vi "test Script EST CD.vi"(8 "error in (no error)":errorcluster, 11 "TestCase in":refnum<class "Scripting API Test Case.lvclass">) -> (0 "error out":errorcluster, 3 "TestCase out":refnum<class "Scripting API Test Case.lvclass">)   [LabVIEW 2015, in "Scripting API Test Case.lvclass"]
uses:
  Scripting API Test Case.lvclass
  Scripting API/Custom Device/Engine Simulation Toolkit Custom Device Settings.ctl
  NationalInstruments.VeriStand.SystemDefinitionAPI
  <userlib>/_OpenG.lib/file/file.llb/Append Path to Root if Relative - Scalar__ogtk.vi
  <vilib>/addons/_JKI Toolkits/VI Tester/TestCase.llb/TestCase.lvclass
  niveristand-custom-device-testing-tools/VeriStandTestUtilities/VeriStandTestUtilities.lvlib
  Scripting API/Engine Simulation Toolkit Scripting API.lvlib
panel:
  in  "Save?":bool
  out "Output Filename":string
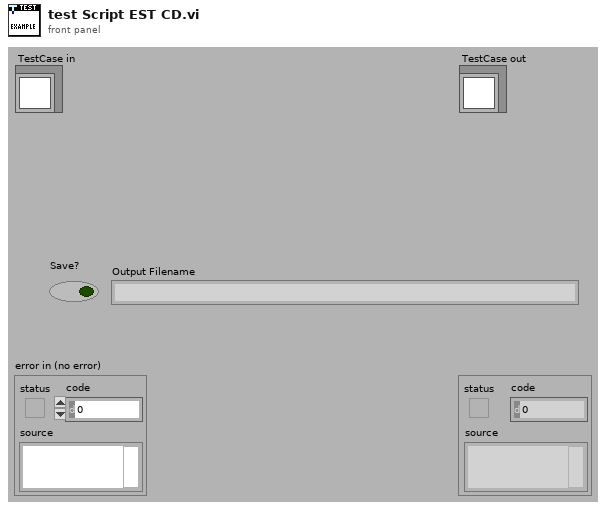
[diagram p1: front panel]
types:
  T1 = typedef "Engine Simulation Toolkit Scripting API.lvlib/Engine Simulation Toolkit Custom Device Settings.ctl" = cluster{"Name":string, "Execution priority":enum16{"Low", "Medium", "High"}, "Rate decimation":i32, "CPU":i32}
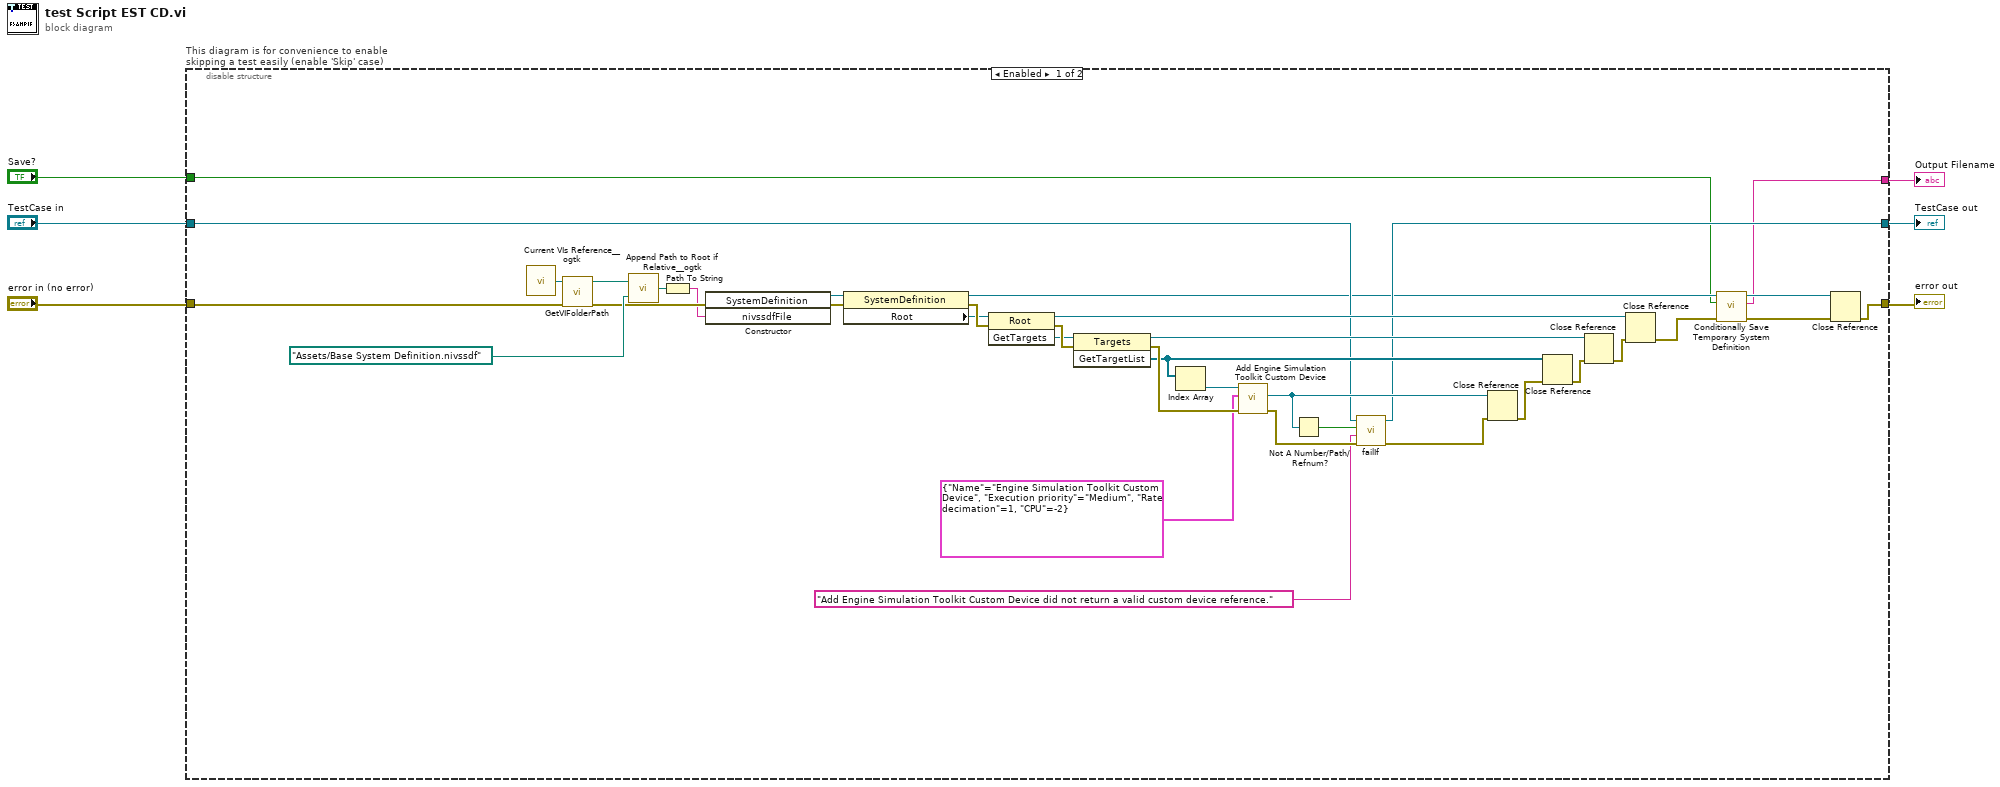
[diagram p0: block diagram]
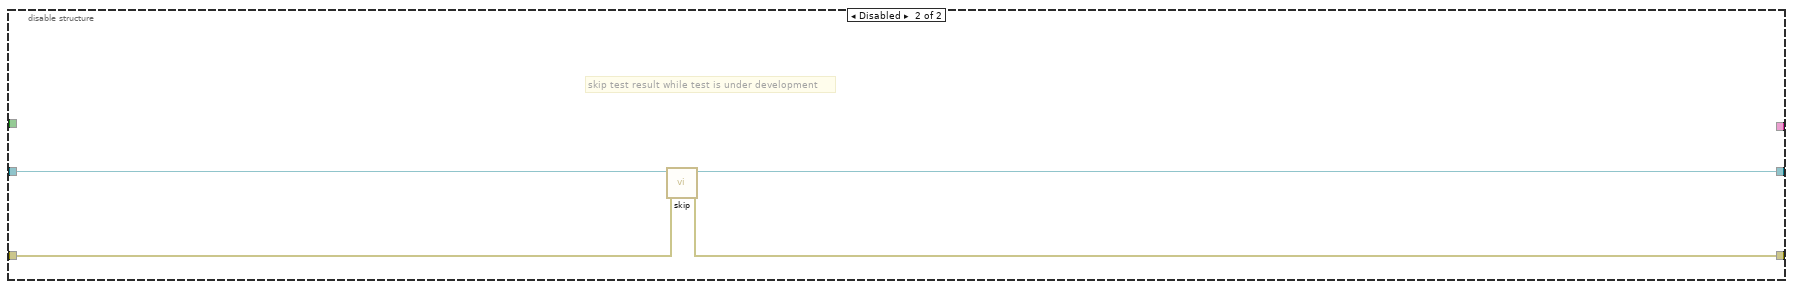
[diagram p2: hidden frame]
diagram:
  n1 = disable-structure "This diagram is for convenience to enable skipping a test easily (enable 'Skip' case)" shown="Enabled" {
    disable-tunnel: "TestCase in" -> [w13 w46]
    disable-tunnel: [w14 w44] -> w3
    disable-tunnel: [w33 w45] -> w5
    disable-tunnel: "error in (no error)" -> [w41 w43]
    disable-tunnel: [w8 _] -> w2
    disable-tunnel: "Save?" -> [w7 _]
    frame Enabled {
      n2 = call <userlib>:"Current VIs Reference__ogtk.vi"() -> ("Current VI's reference"=w42:refnum<vi>)  [unwired: 5 in]
      n3 = call "GetVIFolderPath.vi"("error in (no error)"=w41, "VI Reference in"=w42) -> ("error out"=w37:errorcluster, "VI Folder Path out"=w40:path)  [unwired: 8 in]
      n4 = call-poly <userlib>:"Append Path to Root if Relative__ogtk.vi"("Absolute or Relative Path"=path "Assets/Base System Definition.nivssdf", "Root Path"=w40) -> ("Absolute or Appended Path"=w38:path)
      n5 = Path To String(path=w38) -> (string=w35:string)
      n6 = constructor class="SystemDefinition"(error in=w37, "nivssdfFile"=w35) -> (reference out=w34:refnum<k24>, error out=w36:errorcluster)  [unwired: 2 in, 2 out]
      n7 = property class="SystemDefinition"(reference=w34, error in=w36) -> (reference out=w10:refnum<k24>, error out=w31:errorcluster, "Root"=w30:refnum<k24>)
      n8 = invoke class="Root" method="GetTargets"(reference=w30, error in=w31) -> (reference out=w32:refnum<k24>, error out=w27:errorcluster, "GetTargets"=w26:refnum<k24>)  [unwired: 1 in]
      n9 = invoke class="Targets" method="GetTargetList"(reference=w26, error in=w27) -> (reference out=w28:refnum<k24>, error out=w23:errorcluster, "GetTargetList"=w22:refnum<k24>[])  [unwired: 1 in]
      n10 = Index Array(array=w22) -> (element=w24:refnum<k24>)  [unwired: 1 in]
      n11 = call "Add Engine Simulation Toolkit Custom Device.vi"("error in (no error)"=w23, "Settings"=T1 {"Name"="Engine Simulation Toolkit Custom Device", "Execution priority"=enum."Medium", "Rate decimation"=1, "CPU"=-2} ("Engine Simulation Toolkit Custom Device Settings"), "Target in"=w24) -> ("error out"=w19:errorcluster, "EST Custom Device"=w16:refnum<k24>)  [unwired: 6 in, 1 out]
      n12 = Not A Number/Path/Refnum?(number/path/refnum=w16) -> (NaN/Path/Refnum?=w20:bool)
      n13 = call-dynamic "failIf.vi"("error in (no error)"=w19, "message (\"\")"="Add Engine Simulation Toolkit Custom Device did not return a valid custom device reference." ("message (\"\")"), "fail"=w20, "TestCase in"=w13) -> ("error out"=w15:errorcluster, "TestCase out"=w14:refnum<class "Scripting API Test Case.lvclass">)  [unwired: 6 in]
      n14 = Close Reference(reference=w16, error in (no error)=w15) -> (error out=w17:errorcluster)
      n15 = Close Reference(reference=w22, error in (no error)=w17) -> (error out=w25:errorcluster)
      n16 = Close Reference(reference=w28, error in (no error)=w25) -> (error out=w29:errorcluster)
      n17 = Close Reference(reference=w32, error in (no error)=w29) -> (error out=w9:errorcluster)
      n18 = call "Conditionally Save Temporary System Definition.vi"("error in (no error)"=w9, "Save?"=w7, ".NET Refnum in"=w10) -> ("error out"=w12:errorcluster, "filename"=w8:string, ".NET Refnum out"=w11:refnum<k24>)  [unwired: 6 in]
      n19 = Close Reference(reference=w11, error in (no error)=w12) -> (error out=w33:errorcluster)
    }
    frame Disabled {
      # "skip test result while test is under development"
      n20 = call <vilib>:"skip.vi"("error in (no error)"=w43, "TestCase in"=w46) -> ("error out"=w45:errorcluster, "TestCase out"=w44:refnum<class "Scripting API Test Case.lvclass">)  [unwired: 8 in]
    }
  }
  "error out" <- w5
  "TestCase out" <- w3
  "Output Filename" <- w2
